vi "Post Loop Action.vi"(8 "error in (no error)":errorcluster, 10 "Module Data In":refnum<class "Rename.lvclass">, 11 "Event Registration Refnum":refnum<event-registration>) -> (0 "error out":errorcluster)   [LabVIEW 2015, in "Generic Module Library.lvlib" / "Template G_Module.lvlib"]
uses:
  Template G_Module.lvlib
  Module Class/Rename.lvclass
  Private Controls/Event Item.ctl
  Module Communications/Queue Support/Queue Reference Actions.ctl
  Module Broadcasts/Broadcast Support/Registration Actions.ctl
  Module Broadcasts/Broadcast Support/Broadcast Actions.ctl
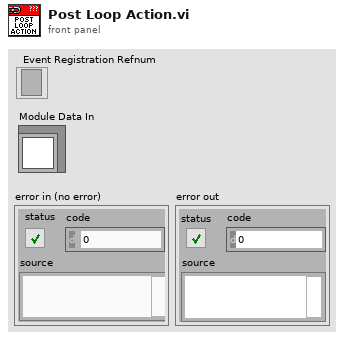
[diagram p1: front panel]
types:
  T1 = typedef "Generic Module Library.lvlib/Template G_Module.lvlib/Broadcast Actions.ctl" = enum16{"Create", "Get", "Destroy"}
  T2 = typedef "Generic Module Library.lvlib/Template G_Module.lvlib/Registration Actions.ctl" = enum16{"Create", "Get", "Destroy"}
  T3 = typedef "Generic Module Library.lvlib/Template G_Module.lvlib/Queue Reference Actions.ctl" = enum16{"Release", "Set", "Get"}
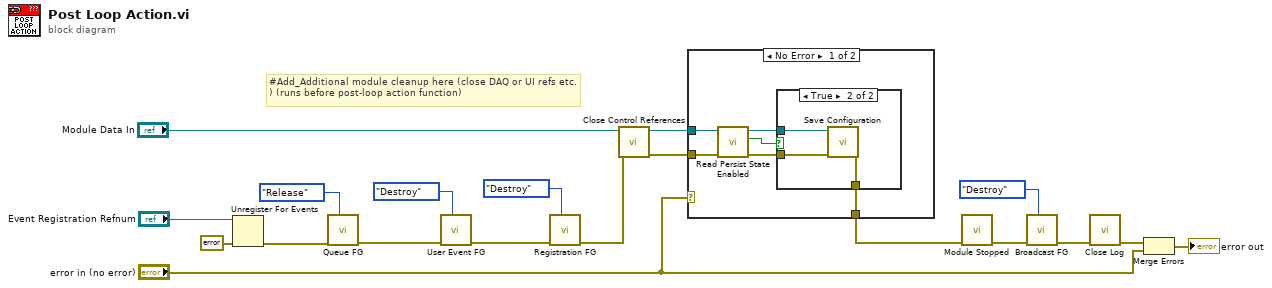
[diagram p0: block diagram]
diagram:
  # "#Add_Additional module cleanup here (close DAQ or UI refs etc.) (runs before post-loop action function)"
  n1 = Unregister For Events(event registration refnum="Event Registration Refnum", error in=errorcluster {"status"=FALSE, "code"=0, "source"=""} ("error in (no error)")) -> (error out=w18:errorcluster)
  n2 = call "Queue FG.vi"("Queue Reference Actions"=Queue_Reference_Actions."Release", "error in"=w18) -> ("error out"=w17:errorcluster)  [unwired: 8 in, 1 out]
  n3 = call "User Event FG.vi"("User Event Actions"=enum16{"Destroy", "Create", "Get"}."Destroy", "error in"=w17) -> ("error out"=w7:errorcluster)  [unwired: 8 in, 1 out]
  n4 = call "Registration FG.vi"("Registration Actions"=Registration_Actions."Destroy", "error in"=w7) -> ("error out"=w9:errorcluster)  [unwired: 8 in, 1 out]
  n5 = call "Close Control References.vi"("error in (no error)"=w9, "Rename in"="Module Data In") -> ("error out"=w11:errorcluster, "Rename out"=w12:refnum<class "Rename.lvclass">)  [unwired: 8 in]
  n6 = case shown="No Error" "error in (no error)" {
    tunnel: w12 -> [w24 _]
    tunnel: w11 -> [w22 w30]
    tunnel: [w25 w30] -> w10
    frame No Error {
      n7 = call-dynamic "Read Persist State Enabled.vi"("error in (no error)"=w22, "Rename in"=w24) -> ("error out"=w21:errorcluster, "Persist State Enabled"=w20:bool, "Rename out"=w23:refnum<class "Rename.lvclass">)  [unwired: 7 in]
      n8 = case shown="True" w20 {
        tunnel: w23 -> [_ w29]
        tunnel: w21 -> [w26 w28]
        tunnel: [w26 w27] -> w25
        frame False {
        }
        frame True {
          n9 = call "Save Configuration.vi"("error in"=w28, "Module Data"=w29) -> ("error out"=w27:errorcluster)  [unwired: 9 in]
        }
      }
    }
    frame Error {
    }
  }
  n10 = call "Module Stopped.vi"("error in"=w10) -> ("error out"=w5:errorcluster)  [unwired: 10 in]
  n11 = call "Broadcast FG.vi"("Broadcast Actions"=Broadcast_Actions."Destroy", "error in"=w5) -> ("error out"=w4:errorcluster)  [unwired: 8 in, 1 out]
  n12 = call "Close Log.vi"("error in"=w4) -> ("error out"=w8:errorcluster)  [unwired: 10 in]
  n13 = Merge Errors(w8, "error in (no error)") -> (→"error out":errorcluster)
